vi "Demo - Custome Node.vi"() -> ()   [LabVIEW 2021]
uses:
  DoublyLinkedList/DoublyLinkedList.lvclass
  CustomeNode/CustomeNode.lvclass
panel:
  out "error out":errorcluster
  out "data":i32[](array[numeric])
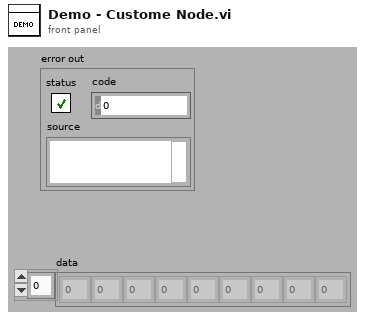
[diagram p1: front panel]
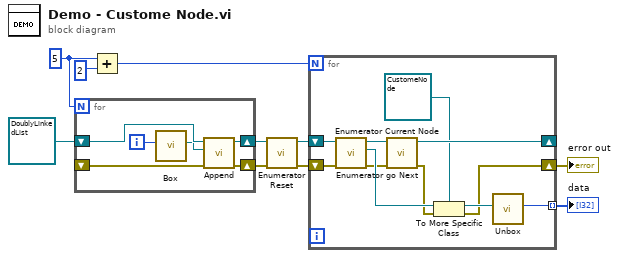
[diagram p0: block diagram]
diagram:
  w9 = 5
  n1 = for {
    N: w9 -> [_]
    shift-right: [w14] -> w6
    shift-left: refnum<class "DoublyLinkedList.lvclass"> refnum ("DoublyLinkedList.lvclass") -> [w15]
    shift-right: [w13] -> w5
    shift-left: _ -> [w12]
    i -> [w16]
    n2 = call "Box.vi"("data"=w16) -> ("CustomeNode out"=w11:refnum<class "CustomeNode.lvclass">)  [unwired: 10 in]
    n3 = call-dynamic "Append.vi"("error in (no error)"=w12, "list node"=w11, "List in"=w15) -> ("error out"=w13:errorcluster, "List out"=w14:refnum<class "DoublyLinkedList.lvclass">)  [unwired: 7 in]
  }
  n4 = Add(x=w9, y=2) -> (x+y=w7:i32)
  n5 = call-dynamic "Enumerator Reset.vi"("error in (no error)"=w5, "List in"=w6) -> ("error out"=w4:errorcluster, "List out"=w3:refnum<class "DoublyLinkedList.lvclass">)  [unwired: 8 in]
  n6 = for {
    N: w7 -> [_]
    shift-right: [w27] -> _
    shift-left: w3 -> [w25]
    shift-right: [w17] -> w10
    shift-left: w4 -> [w24]
    tunnel: [w18] -> w2 mode=indexing
    n7 = call-dynamic "Enumerator Current Node.vi"("error in (no error)"=w24, "List in"=w25) -> ("error out"=w21:errorcluster, "Node"=w22:refnum<class "ListNode.lvclass">, "List out"=w26:refnum<class "DoublyLinkedList.lvclass">)  [unwired: 7 in]
    n8 = call-dynamic "Enumerator go Next.vi"("error in (no error)"=w21, "List in"=w26) -> ("error out"=w20:errorcluster, "List out"=w27:refnum<class "DoublyLinkedList.lvclass">)  [unwired: 8 in]
    n9 = To More Specific Class(target class=refnum<class "CustomeNode.lvclass"> refnum ("CustomeNode.lvclass"), reference=w22, error in=w20) -> (specific class reference=w19:refnum<class "CustomeNode.lvclass">, error out=w17:errorcluster)
    n10 = call "Unbox.vi"("CustomeNode in"=w19) -> ("data"=w18:i32)  [unwired: 10 in]
  }
  "data" <- w2
  "error out" <- w10
